vi "ILABR_GetVI.vi"(2 "port":i32, 3 "machineName":string, 4 "path":string) -> (0 "errorOut":string, 1 "viReference":refnum<vi>)   [LabVIEW 2009]
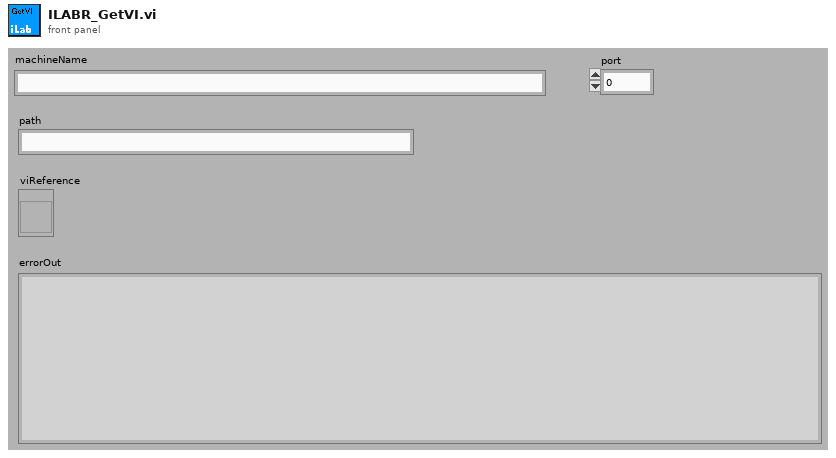
[diagram p1: front panel]
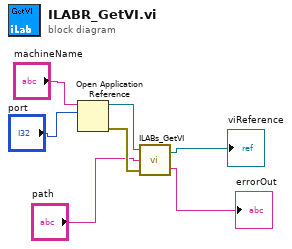
[diagram p0: block diagram]
diagram:
  n1 = Open Application Reference(10:"port", 11:"machineName") -> (0:w6:errorcluster, 3:w7:refnum<vi>)  [unwired: 1 in, 1 out]
  n2 = call "ILABs_GetVI.vi"("errorIn"=w6, "path"="path", "appReference"=w7) -> ("errorOut"=→"errorOut":string, "vi reference"=→"viReference":refnum<vi>)
